vi "글꼴설정.vi"() -> ()   [LabVIEW 2014]
uses:
  System.Windows.Forms
  System.Drawing
panel:
  out "Color":u32(colorbox) caption="색"
  out "Name":string
  out "Size":sgl
  out "ShowDialog":i32(ring) items=["None", "OK", "Cancel", "Abort", "Retry", "Ignore", "Yes", "No"]
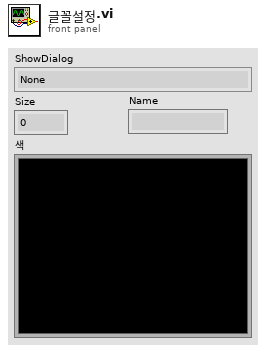
[diagram p1: front panel]
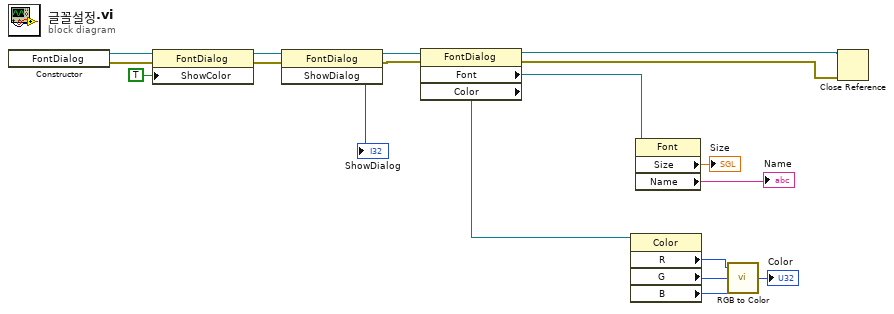
[diagram p0: block diagram]
diagram:
  n1 = constructor class="FontDialog"() -> (reference out=w18:refnum<k24>, error out=w17:errorcluster)  [unwired: 3 in, 1 out]
  n2 = property class="FontDialog"(reference=w18, error in=w17, "ShowColor"=TRUE) -> (reference out=w15:refnum<k24>, error out=w14:errorcluster)
  n3 = invoke class="FontDialog" method="ShowDialog"(reference=w15, error in=w14) -> (reference out=w12:refnum<k24>, error out=w11:errorcluster, "ShowDialog"=→"ShowDialog":i32)  [unwired: 1 in]
  n4 = property class="FontDialog"(reference=w12, error in=w11) -> (reference out=w10:refnum<k24>, error out=w9:errorcluster, "Font"=w8:refnum<k24>, "Color"=w5:refnum<k24>)
  n5 = property class="Color"(reference=w5) -> ("R"=w4:u8, "G"=w3:u8, "B"=w2:u8)  [unwired: 1 in, 2 out]
  n6 = property class="Font"(reference=w8) -> ("Size"=→"Size":sgl, "Name"=→"Name":string)  [unwired: 1 in, 2 out]
  n7 = call <vilib>:"RGB to Color.vi"("B"=w2, "G"=w3, "R"=w4) -> ("Color"=→"Color":u32)
  n8 = Close Reference(reference=w10, error in (no error)=w9) -> ()  [unwired: 1 out]
